vi "rsp_New Pumps Data.vi"(4 "Show in Debugger?":bool=TRUE, 6 "Message Priority":T1=enum."Normal", 8 "error in":errorcluster, 10 "Data in":T2={"Насос"={"Давление заданное"=0.3, "Давление MAX заданное"=100.0, "Давление в насосе"=0.0, "Давление в системе"=99.99, "Расход заданый"=0.0, "Расход текущий"=0.0, "Объём заданный"=0.0, "Объём текущий"=0.0, "Позиция насоса %"=0.0, "Ток двигателя"=0.0, "controlMsg"="", "Клапан k_sys"=FALSE, "Клапан k_res"=FALSE, "Клапан k_air"=FALSE, "Вверх"=FALSE, "Домой"=FALSE, "Вниз"=FALSE, "Старт расход"=FALSE, "Старт давление"=FALSE, "Сброс объёма"=FALSE, "Сброс давления Рсис"=FALSE, "Сброс давления Рнас"=FALSE, "Bits"={"plc_control"=FALSE, "lag_control"=FALSE, "mstop_control"=FALSE, "st_home"=FALSE, "error"=FALSE, "mstart"=FALSE, "pair"=FALSE, "startQ"=FALSE, "startP"=FALSE, "volume_Stop"=FALSE}}, "Насос 2"={"Давление заданное"=0.3, "Давление MAX заданное"=100.0, "Давление в насосе"=0.0, "Давление в системе"=99.99, "Расход заданый"=0.0, "Расход текущий"=0.0, "Объём заданный"=0.0, "Объём текущий"=0.0, "Позиция насоса %"=0.0, "Ток двигателя"=0.0, "controlMsg"="", "Клапан k_sys"=FALSE, "Клапан k_res"=FALSE, "Клапан k_air"=FALSE, "Вверх"=FALSE, "Домой"=FALSE, "Вниз"=FALSE, "Старт расход"=FALSE, "Старт давление"=FALSE, "Сброс объёма"=FALSE, "Сброс давления Рсис"=FALSE, "Сброс давления Рнас"=FALSE, "Bits"={"plc_control"=FALSE, "lag_control"=FALSE, "mstop_control"=FALSE, "st_home"=FALSE, "error"=FALSE, "mstart"=FALSE, "pair"=FALSE, "startQ"=FALSE, "startP"=FALSE, "volume_Stop"=FALSE}}, "Насосная система"={"Давление заданное"=0.3, "Давление в системе"=99.99, "Расход заданый"=0.0, "Расход текущий"=0.0, "Объём заданный"=0.0, "Объём текущий"=0.0, "Старт давление"=FALSE, "Старт расход"=FALSE, "Сброс объёма"=FALSE, "plc_control"=FALSE, "lag_control"=FALSE, "mstop_control"=FALSE, "Давление"={"АЦП CH 0"=0.0, "АЦП CH 1"=0.0, "АЦП CH 2"=0.0, "АЦП CH 3"=0.0, "АЦП CH 4"=0.0, "АЦП CH 5"=0.0, "АЦП CH 6"=0.0, "АЦП CH 7"=0.0}, "Modbus"={"Массив чтения"=[], "Массив записи"=[]}}} {"Насосная система"."Давление"."АЦП CH 7" format="%.3f"; "Насосная система"."Давление"."АЦП CH 6" format="%.3f"; "Насосная система"."Давление"."АЦП CH 5" format="%.3f"; "Насосная система"."Давление"."АЦП CH 4" format="%.3f"; "Насосная система"."Давление"."АЦП CH 3" format="%.3f"; "Насосная система"."Давление"."АЦП CH 2" format="%.3f"; "Насосная система"."Давление"."АЦП CH 1" format="%.3f"; "Насосная система"."Давление"."АЦП CH 0" format="%.3f"; "Насосная система"."Объём текущий" min=0.0 max=9999.0 step=0.0001 format="%#_4f"; "Насосная система"."Объём заданный" min=0.0 max=9999.0 step=0.0001 format="%#_5f"; "Насосная система"."Расход текущий" format="%#_4f"; "Насосная система"."Расход заданый" min=-150.0 max=150.0 step=0.0001 format="%#_5f"; "Насосная система"."Давление в системе" format="%.2f"; "Насосная система"."Давление заданное" min=0.3 max=100.0 step=0.01 format="%#_5f"; "Насос 2"."Ток двигателя" format="%#_5f"; "Насос 2"."Расход текущий" format="%#_4f"; "Насос 2"."Давление в системе" format="%.2f"; "Насос 2"."Объём текущий" min=0.0 max=9999.0 step=0.0001 format="%#_4f"; "Насос 2"."Объём заданный" min=0.0 max=9999.0 step=0.0001 format="%#_5f"; "Насос 2"."Давление MAX заданное" min=0.0 max=100.0 step=0.01 format="%#_5f"; "Насос 2"."Давление заданное" min=0.3 max=100.0 step=0.01 format="%#_5f"; "Насос 2"."Расход заданый" min=-150.0 max=150.0 step=0.0001 format="%#_5f"; "Насос 2"."Давление в насосе" format="%.3f"; "Насос 2"."Позиция насоса %" scale=0.0..100.0 scale format="%.2f"; "Насос"."Ток двигателя" format="%#_5f"; "Насос"."Расход текущий" format="%#_4f"; "Насос"."Давление в системе" format="%.2f"; "Насос"."Объём текущий" min=0.0 max=9999.0 step=0.0001 format="%#_4f"; "Насос"."Объём заданный" min=0.0 max=9999.0 step=0.0001 format="%#_5f"; "Насос"."Давление MAX заданное" min=0.0 max=100.0 step=0.01 format="%#_5f"; "Насос"."Давление заданное" min=0.3 max=100.0 step=0.01 format="%#_5f"; "Насос"."Расход заданый" min=-150.0 max=150.0 step=0.0001 format="%#_5f"; "Насос"."Давление в насосе" format="%.3f"; "Насос"."Позиция насоса %" scale=0.0..100.0 scale format="%.2f"}, 11 "Pumps Worker in":refnum<class "Pumps Worker.lvclass">) -> (0 "error out":errorcluster, 3 "dup Pumps Worker out":refnum<class "Pumps Worker.lvclass">)   [LabVIEW 2023, in "pump_Lib.lvlib" / "Pumps Worker.lvclass"]
doc: "This VI sends a <b>Public API Response</b> message to a registered MHL case of the Caller of the Worker that owns this VI.\n---\nWorkers Public API Response"
uses:
  Pumps Worker.lvclass
  C:/Program Files/National Instruments/LabVIEW 2023/vi.lib/addons/_Workers/Library/Classes/Worker/Worker.lvclass
  rsp_New Pumps Data.ctl
  TypeDef/pump_Type_Pair_L.ctl
  TypeDef/pump_Type_Pair_R.ctl
  TypeDef/pair_Type.ctl
  <vilib>/addons/_Workers/Library/Classes/Message/Priority.ctl
  Pumps Worker.lvclass/Pumps Worker.ctl
  <vilib>/Utility/error.llb/Error Cluster From Error Code.vi
  <vilib>/addons/_Workers/Library/Classes/Worker/Worker.lvclass
  <vilib>/addons/_Workers/Library/Classes/Message Queue/Message Queue.lvclass
  <vilib>/ErrorRing/Error Ring.xnode
  <vilib>/addons/_Workers/Library/Classes/Message/Message.lvclass
  pump_Lib.lvlib
panel:
  # "%"
  # "%"
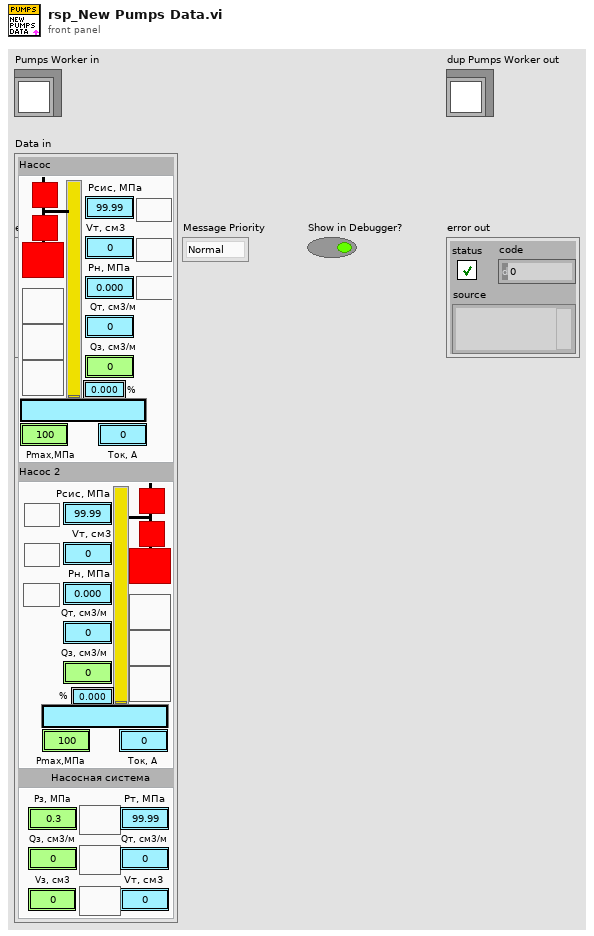
[diagram p1: front panel]
types:
  T1 = typedef "Workers.lvlib/Message.lvclass/Priority.ctl" = enum16{"Low", "Normal", "High"}
  T2 = typedef "pump_Lib.lvlib/Pumps Worker.lvclass/rsp_New Pumps Data.ctl" = cluster{"Насос":T3, "Насос 2":T4, "Насосная система":T5}
  T3 = typedef "pump_Lib.lvlib/pump_Type_Pair_L.ctl" = cluster{"Давление заданное":dbl, "Давление MAX заданное":dbl, "Давление в насосе":dbl, "Давление в системе":dbl, "Расход заданый":dbl, "Расход текущий":dbl, "Объём заданный":dbl, "Объём текущий":dbl, "Позиция насоса %":dbl, "Ток двигателя":dbl, "controlMsg":string, "Клапан k_sys":bool, "Клапан k_res":bool, "Клапан k_air":bool, "Вверх":bool, "Домой":bool, "Вниз":bool, "Старт расход":bool, "Старт давление":bool, "Сброс объёма":bool, "Сброс давления Рсис":bool, "Сброс давления Рнас":bool, "Bits":cluster{"plc_control":bool, "lag_control":bool, "mstop_control":bool, "st_home":bool, "error":bool, "mstart":bool, "pair":bool, "startQ":bool, "startP":bool, "volume_Stop":bool}}
  T4 = typedef "pump_Lib.lvlib/pump_Type_Pair_R.ctl" = cluster{"Давление заданное":dbl, "Давление MAX заданное":dbl, "Давление в насосе":dbl, "Давление в системе":dbl, "Расход заданый":dbl, "Расход текущий":dbl, "Объём заданный":dbl, "Объём текущий":dbl, "Позиция насоса %":dbl, "Ток двигателя":dbl, "controlMsg":string, "Клапан k_sys":bool, "Клапан k_res":bool, "Клапан k_air":bool, "Вверх":bool, "Домой":bool, "Вниз":bool, "Старт расход":bool, "Старт давление":bool, "Сброс объёма":bool, "Сброс давления Рсис":bool, "Сброс давления Рнас":bool, "Bits":cluster{"plc_control":bool, "lag_control":bool, "mstop_control":bool, "st_home":bool, "error":bool, "mstart":bool, "pair":bool, "startQ":bool, "startP":bool, "volume_Stop":bool}}
  T5 = typedef "pump_Lib.lvlib/pair_Type.ctl" = cluster{"Давление заданное":dbl, "Давление в системе":dbl, "Расход заданый":dbl, "Расход текущий":dbl, "Объём заданный":dbl, "Объём текущий":dbl, "Старт давление":bool, "Старт расход":bool, "Сброс объёма":bool, "plc_control":bool, "lag_control":bool, "mstop_control":bool, "Давление":cluster{"АЦП CH 0":dbl, "АЦП CH 1":dbl, "АЦП CH 2":dbl, "АЦП CH 3":dbl, "АЦП CH 4":dbl, "АЦП CH 5":dbl, "АЦП CH 6":dbl, "АЦП CH 7":dbl}, "Modbus":cluster{"Массив чтения":u16[], "Массив записи":u16[]}}
  T6 = typedef "Workers.lvlib/Case Label.ctl" = string
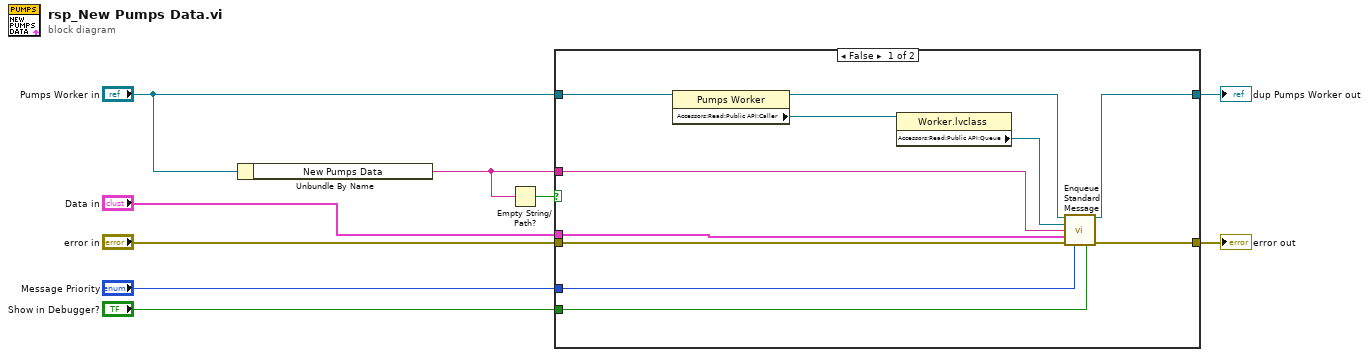
[diagram p0: block diagram]
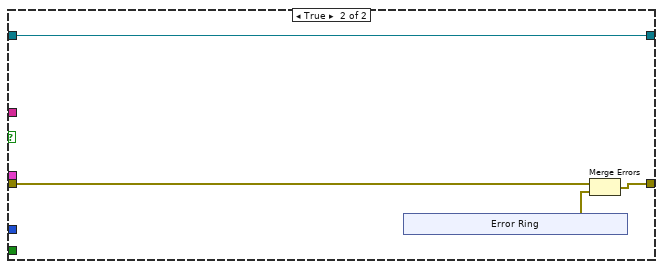
[diagram p2: hidden frame]
diagram:
  n1 = Unbundle By Name("Pumps Worker in") -> ("New Pumps Data"=w4:T6)
  n2 = Empty String/Path?(string/path=w4) -> (empty?=w5:bool)
  n3 = case shown="False" w5 {
    tunnel: "error in" -> [w20 w21]
    tunnel: [w19 w22] -> w8
    tunnel: "Data in" -> [w16 _]
    tunnel: [w18 w24] -> w6
    tunnel: "Pumps Worker in" -> [w13 w24]
    tunnel: w4 -> [w17 _]
    tunnel: "Show in Debugger?" -> [w15 _]
    tunnel: "Message Priority" -> [w14 _]
    frame False {
      n4 = property class="Pumps Worker"(reference=w13) -> (reference out=w12:refnum<class "Pumps Worker.lvclass">, "Accessors:Read:Public API:Caller"=w10:refnum<class "Worker.lvclass">)  [unwired: 1 in, 1 out]
      n5 = property class="Worker.lvclass"(reference=w10) -> ("Accessors:Read:Public API:Queue"=w11:refnum<class "Message Queue.lvclass">)  [unwired: 1 in, 2 out]
      n6 = call-dynamic "Enqueue Standard Message.vi"("Worker"=w12, "Message Queue"=w11, "Case Label"=w17, "Data"=w16, "error in (no error)"=w20, "Priority (Normal)"=w14, "Send Message to Debugger? (T)"=w15) -> ("dup Worker out"=w18:refnum<class "Pumps Worker.lvclass">, "error out"=w19:errorcluster)  [unwired: 7 in]
    }
    frame True {
      n7 = xnode "Error Ring"() -> ("error out"=w23:errorcluster)
      n8 = Merge Errors(w21, w23) -> (w22:errorcluster)
    }
  }
  "error out" <- w8
  "dup Pumps Worker out" <- w6
